vi "FIR filter neu.vi"(0 "order":i32=2, 4 "filter type":T1(ring), 6 "higher pass freq":dbl=0.4000000000000001 format="%.2f", 7 "lower pass freq":dbl=0.2 format="%.2f", 8 "sampling freq: fs":dbl=1.0 format="%.2f", 9 "3D Unfiltered Data":dbl[][](array[numeric]) format="%.2f") -> (1 "Output Array":dbl[][](graph))   [LabVIEW 2014, in "comm.lvlib"]
uses:
  comm.lvlib
  <vilib>/Analysis/NI_AALBase.lvlib
  <vilib>/ptbypt/NI_PtbyPt.lvlib
panel:
  # "Copyright Americo A. Migliaccio (c) 2002 All Rights Reserved by Author"
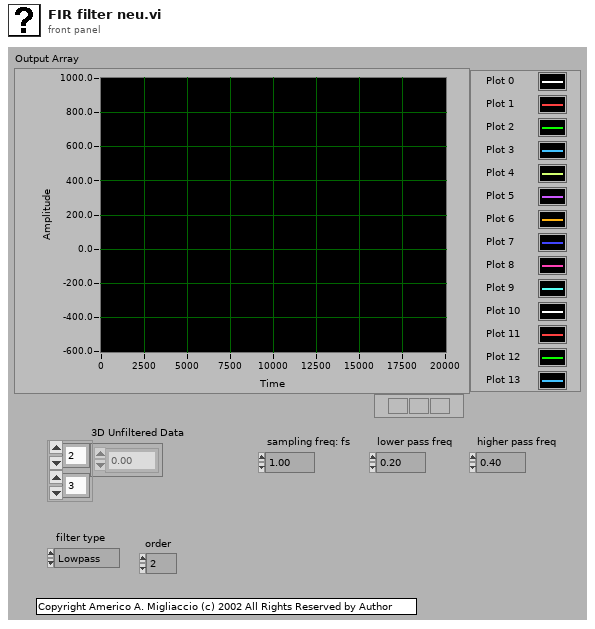
[diagram p1: front panel]
types:
  T1 = enum32{"Lowpass", "Highpass", "Bandpass", "Bandstop"}
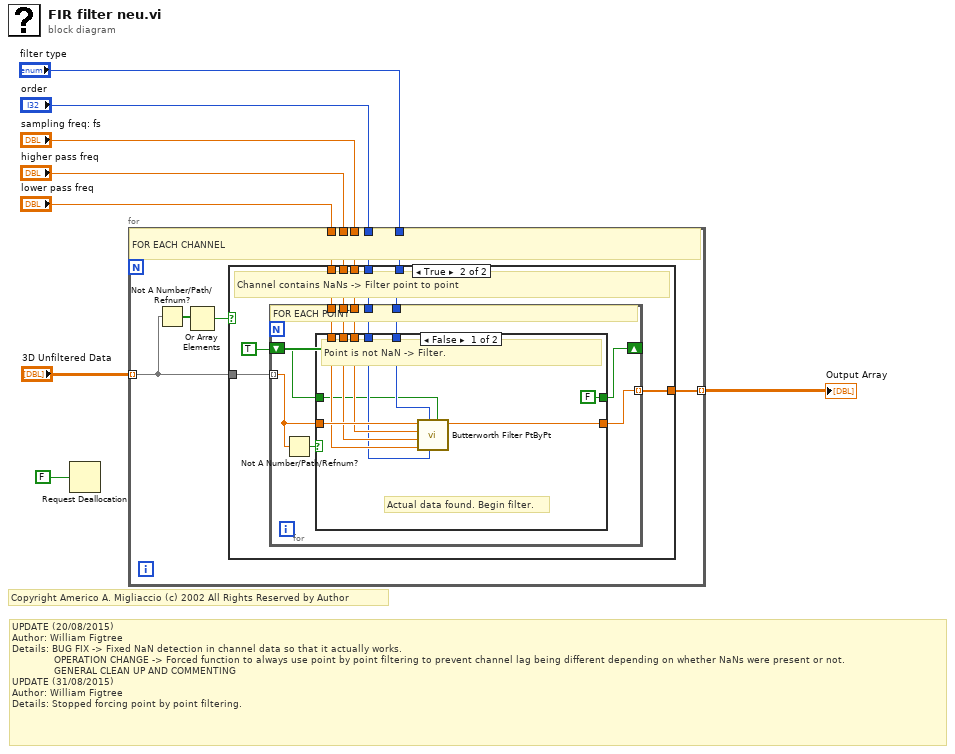
[diagram p0: block diagram]
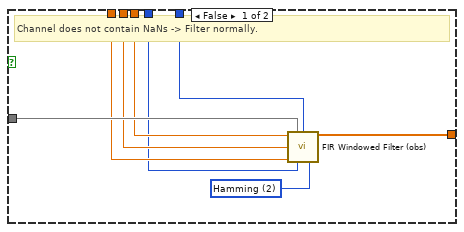
[diagram p2: hidden frame]
diagram:
  # "UPDATE (20/08/2015)\nAuthor: William Figtree\nDetails: BUG FIX -> Fixed NaN detection in channel data so that it actually works.\n              OPERATION CHANGE -> Forced function to always use point by point filtering to prevent channel lag being different depending on whether NaNs were present or not.\n              GENERAL CLEAN UP AND COMMENTING\nUPDATE (31/08/2015)\nAuthor: William Figtree\nDetails: Stopped forcing point by point filtering."
  # "Copyright Americo A. Migliaccio (c) 2002 All Rights Reserved by Author"
  n1 = Request Deallocation(FALSE ("flag")) -> ()
  n2 = for {
    tunnel: "sampling freq: fs" -> [w17]
    tunnel: "higher pass freq" -> [w16]
    tunnel: "lower pass freq" -> [w15]
    tunnel: "3D Unfiltered Data" -> [w11] mode=indexing
    tunnel: [w12] -> w5 mode=indexing
    tunnel: "filter type" -> [w14]
    tunnel: "order" -> [w13]
    # "FOR EACH CHANNEL"
    n3 = Not A Number/Path/Refnum?(number/path/refnum=w11) -> (NaN/Path/Refnum?=w9:bool[])
    n4 = Or Array Elements(Boolean array=w9) -> (logical OR=w10:bool)
    n5 = case shown="True" w10 {
      tunnel: w17 -> [w22 w32]
      tunnel: w16 -> [w20 w31]
      tunnel: w15 -> [w21 w30]
      tunnel: w14 -> [w24 w28]
      tunnel: w13 -> [w19 w29]
      tunnel: [w25 w26] -> w12
      tunnel: w11 -> [w23 w33]
      frame False {
        w18 = 2 items=["None", "Hanning", "Hamming", "Triangular", "Blackman", "Exact Blackman", "Blackman-Harris", "Kaiser-Bessel", "Flat Top"] ("window")
        # "Channel does not contain NaNs -> Filter normally."
        n6 = call <vilib>:"FIR Windowed Filter (obs).vi"("sampling freq: fs"=w22, "X"=w23, "filter type"=w24, "low cutoff freq: fl"=w20, "high cutoff freq: fh"=w21, "taps"=w19, "window"=w18) -> ("Filtered X"=w25:dbl[])  [unwired: 7 in, 1 out]
      }
      frame True {
        # "Channel contains NaNs -> Filter point to point"
        n7 = for {
          tunnel: w33 -> [w36] mode=indexing
          tunnel: w32 -> [w43]
          tunnel: w31 -> [w42]
          tunnel: w30 -> [w41]
          tunnel: w29 -> [w40]
          tunnel: w28 -> [w39]
          shift-right: [w34] -> _
          shift-left: TRUE -> [w38]
          tunnel: [w37] -> w26 mode=indexing
          # "FOR EACH POINT"
          n8 = Not A Number/Path/Refnum?(number/path/refnum=w36) -> (NaN/Path/Refnum?=w35:bool)
          n9 = case shown="False" w35 {
            tunnel: w36 -> [w52 w54]
            tunnel: w43 -> [w51 _]
            tunnel: w42 -> [w50 _]
            tunnel: w41 -> [w49 _]
            tunnel: w40 -> [w48 _]
            tunnel: w39 -> [w47 _]
            tunnel: w38 -> [w46 w53]
            tunnel: [w45 w54] -> w37
            tunnel: [FALSE w53] -> w34
            frame False {
              # "Actual data found. Begin filter."
              # "Point is not NaN -> Filter."
              n10 = call <vilib>:"Butterworth Filter PtByPt.vi"("initialize"=w46, "order"=w48, "filter type"=w47, "low cutoff freq: fl"=w49, "high cutoff freq: fh"=w50, "sampling freq: fs"=w51, "x"=w52) -> ("Filtered x"=w45:dbl)  [unwired: 2 in, 1 out]
            }
            frame True {
              # "Point is NaN -> Pass through."
            }
          }
        }
      }
    }
  }
  "Output Array" <- w5
